vi "Example 1.vi"() -> ()   [LabVIEW 2016]
panel:
  out "Image":T1(plugin-control)
  in  "Reading":bool
  in  "Table":i32(listbox)
  in  "Polling Time":i32=50
  in  "Connect":bool
  in  "Remote Port":u16=51236
  in  "IP Address":string="192.168.3.100"
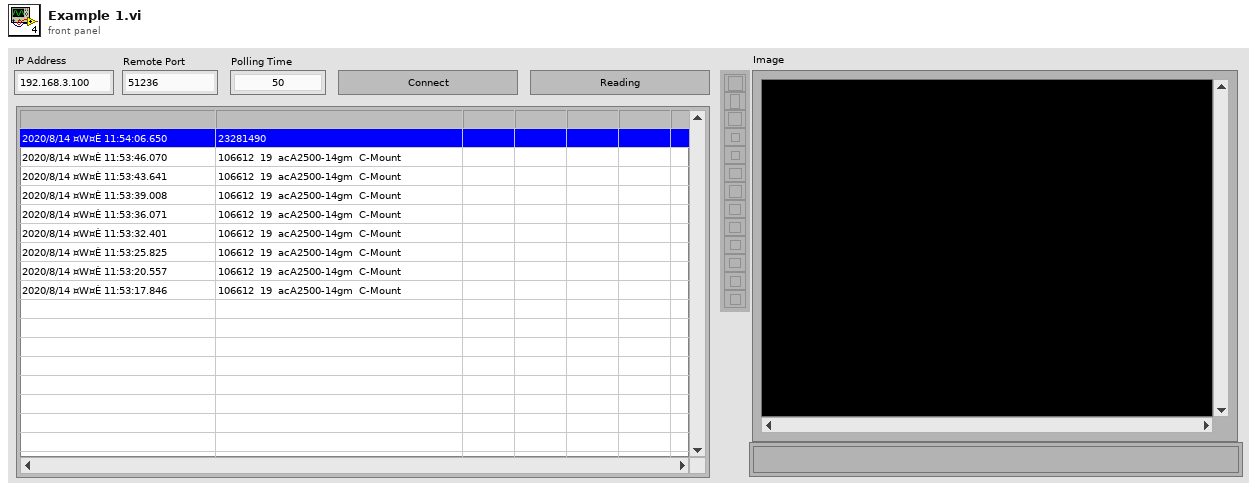
[diagram p1: front panel]
types:
  T1 = typedef "IMAQ Image.ctl" = refnum<image>
  T2 = typedef "Loop Data.ctl" = cluster{"VI Refnum":refnum<vi>, "Timeout":i32, "Code Data":cluster{"Time":timestamp, "Code Data":string}[], "Buffer Data":T3, "Timer":u32, "Image":T1}
  T3 = typedef "Com_Matrix220_Buffer Data.ctl" = cluster{"Connection ID":refnum<k5>}
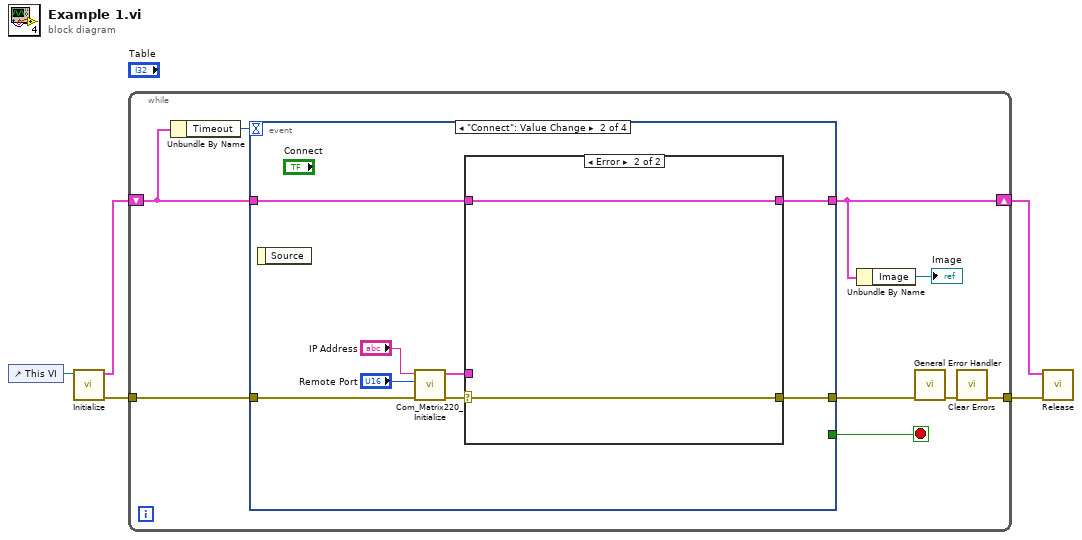
[diagram p0: block diagram]
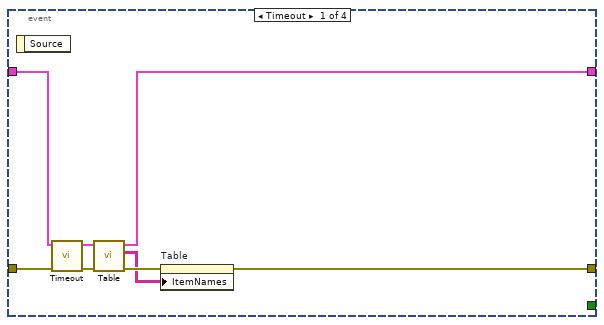
[diagram p2: hidden frame]
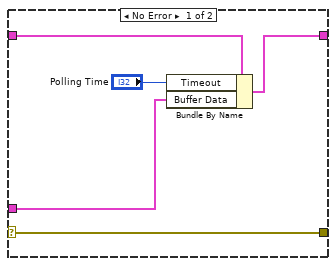
[diagram p3: hidden frame]
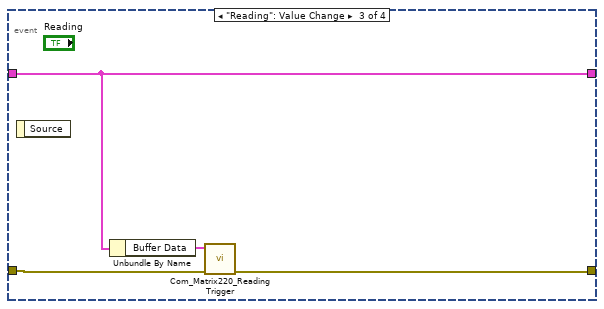
[diagram p4: hidden frame]
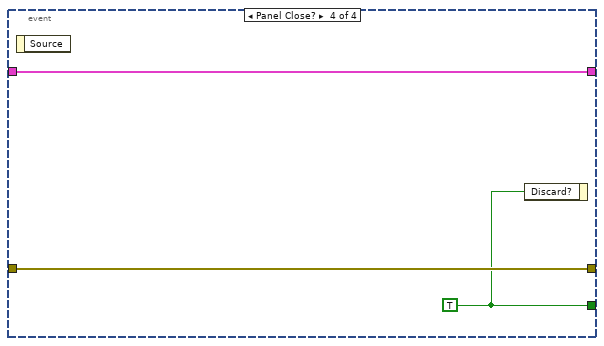
[diagram p5: hidden frame]
diagram:
  n1 = control-ref of="This VI"() -> (w5:refnum<vi>)
  n2 = call "Initialize.vi"("VI Refnum"=w5) -> ("error out"=w4:errorcluster, "Loop Data"=w3:T2)  [unwired: 9 in]
  n3 = while {
    tunnel: w4 -> [w12]
    shift-right: [w7] -> w1
    shift-left: w3 -> [w13]
    tunnel: [w8] -> w2
    stop <- w11 stop-if-true
    n4 = Unbundle By Name(w13) -> ("Timeout"=w14:i32)
    n5 = event shown="[1] \"Connect\": Value Change" {
      selector: _ -> [_ _ _ _]
      dyn-events: _ -> [_ _ _ _]
      timeout: w14 -> [_ _ _ _]
      tunnel: w13 -> [w21 w26 w38 w44]
      tunnel: [w15 w24 w38 w44] -> w7
      tunnel: w12 -> [w22 w30 w41 w43]
      tunnel: [w16 w23 w39 w43] -> w10
      tunnel: [_ _ _ w42] -> w11
      event Timeout {
        n6 = event-data() -> ()  [unwired: 1 in, 1 out]
        n7 = call "Timeout.vi"("error in"=w22, "Loop Data In"=w21) -> ("error out"=w19:errorcluster, "Loop Data Out"=w20:T2)  [unwired: 8 in]
        n8 = call "Table.vi"("error in"=w19, "Loop Data In"=w20) -> ("error out"=w18:errorcluster, "Table"=w17:string[][], "Loop Data Out"=w15:T2)  [unwired: 7 in]
        n9 = property on="Table" class="MCListbox (strict)"(error in=w18, "ItemNames"=w17) -> (error out=w16:errorcluster)  [unwired: 1 in, 1 out]
      }
      event "Connect": Value Change {
        n10 = event-data() -> ()  [unwired: 1 in, 1 out]
        n11 = call "Com_Matrix220_Initialize.vi"("error in"=w30, "Remote Port"="Remote Port", "IP Address"="IP Address") -> ("error out"=w27:errorcluster, "Buffer Data"=w25:T3)  [unwired: 7 in]
        n12 = case shown="Error" w27 {
          selector: w27 -> [w32 w37]
          tunnel: w26 -> [w35 w36]
          tunnel: w25 -> [w34 _]
          tunnel: [w33 w36] -> w24
          tunnel: [w32 w37] -> w23
          frame No Error {
            n13 = Bundle By Name(cluster=w35, "Timeout"="Polling Time", "Buffer Data"=w34) -> (w33:T2)
          }
          frame Error {
          }
        }
      }
      event "Reading": Value Change {
        n14 = event-data() -> ()  [unwired: 1 in, 1 out]
        n15 = Unbundle By Name(w38) -> ("Buffer Data"=w40:T3)
        n16 = call "Com_Matrix220_Reading Trigger.vi"("error in"=w41, "Buffer Data In"=w40) -> ("error out"=w39:errorcluster)  [unwired: 8 in, 1 out]
      }
      event Panel Close? {
        w42 = TRUE
        n17 = event-data() -> ()  [unwired: 1 in, 1 out]
        n18 = event-data("Discard?"=w42) -> ()  [unwired: 1 in, 1 out]
      }
    }
    n19 = Unbundle By Name(w7) -> ("Image"=→"Image":T1)
    n20 = call <vilib>:"General Error Handler.vi"("error in (no error)"=w10) -> ("error out"=w9:errorcluster)  [unwired: 10 in, 4 out]
    n21 = call <vilib>:"Clear Errors.vi"("error in (no error)"=w9) -> ("error out"=w8:errorcluster)  [unwired: 5 in, 1 out]
  }
  n22 = call "Release.vi"("error in"=w2, "Loop Data"=w1) -> ()  [unwired: 9 in, 1 out]
